vi "Autosampler Priming Settings Dialog.vi"(8 "error in":errorcluster, 10 "Valve Pos Names":string[](array[string])) -> (0 "error out":errorcluster, 1 "Cancelled?":bool, 2 "Result":T1)   [LabVIEW 2023]
panel:
  in  "Output Valve Position":u16(ring)=1 items=["1. Needle port", "2. Waste", "3. Disconnected", "4. Disconnected", "5. Disconnected", "6. Water"]
  in  "Input Valve Position":u16(ring)=5 items=["1. Needle port", "2. Waste", "3. Disconnected", "4. Disconnected", "5. Disconnected", "6. Water"]
  in  "Cancel":bool caption="Boolean 2"
  in  "Ok":bool caption="Boolean"
  in  "Number of Cycles":u16=3 min=1 step=1
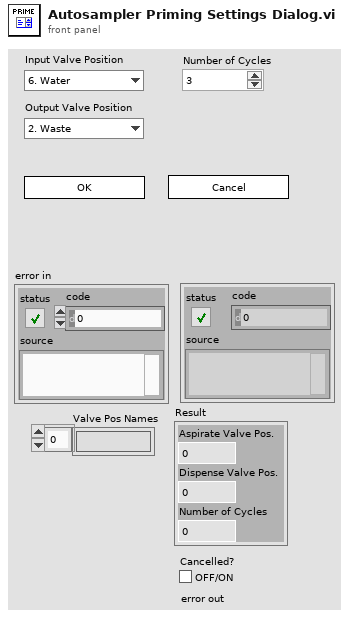
[diagram p1: front panel]
types:
  T1 = cluster{"Aspirate Valve Pos.":u16, "Dispense Valve Pos.":u16, "Number of Cycles":u16}
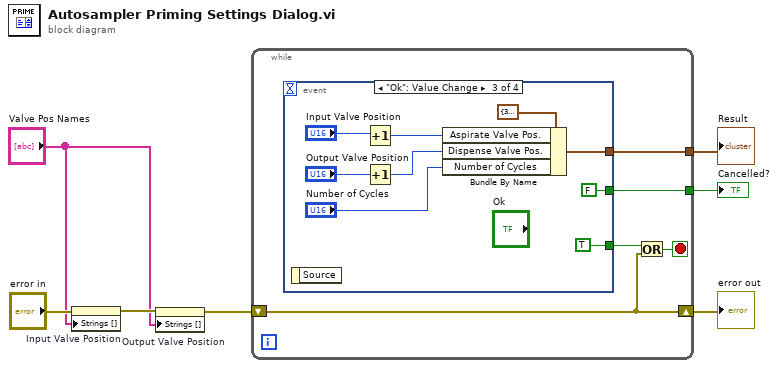
[diagram p0: block diagram]
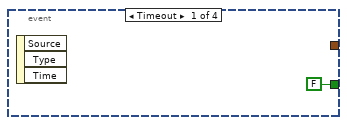
[diagram p2: hidden frame]
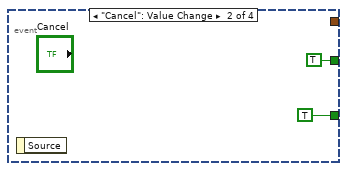
[diagram p3: hidden frame]
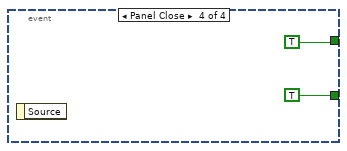
[diagram p4: hidden frame]
diagram:
  n1 = property on="Input Valve Position" class="Ring (strict)"(error in="error in", "Strings []"="Valve Pos Names") -> (error out=w3:errorcluster)  [unwired: 1 in, 1 out]
  n2 = property on="Output Valve Position" class="Ring (strict)"(error in=w3, "Strings []"="Valve Pos Names") -> (error out=w2:errorcluster)  [unwired: 1 in, 1 out]
  n3 = while {
    shift-right: [w8] -> w7
    shift-left: w2 -> [w8]
    tunnel: [w12] -> w6
    tunnel: [w11] -> w5
    stop <- w10 stop-if-true
    n4 = event shown="[2] \"Ok\": Value Change" {
      selector: _ -> [_ _ _ _]
      dyn-events: _ -> [_ _ _ _]
      timeout: _ -> [_ _ _ _]
      tunnel: [FALSE TRUE FALSE TRUE] -> w12
      tunnel: [_ _ w21 _] -> w11
      tunnel: [_ TRUE TRUE TRUE] -> w9
      event Timeout {
        n5 = event-data() -> ()  [unwired: 1 in, 3 out]
      }
      event "Cancel": Value Change {
        n6 = event-data() -> ()  [unwired: 1 in, 1 out]
      }
      event "Ok": Value Change {
        n7 = event-data() -> ()  [unwired: 1 in, 1 out]
        n8 = Increment(x="Input Valve Position") -> (x+1=w18:u16)
        n9 = Increment(x="Output Valve Position") -> (x+1=w16:u16)
        n10 = Bundle By Name(cluster=T1 {"Aspirate Valve Pos."=3, "Dispense Valve Pos."=2, "Number of Cycles"=5}, "Aspirate Valve Pos."=w18, "Dispense Valve Pos."=w16, "Number of Cycles"="Number of Cycles") -> (w21:T1)
      }
      event Panel Close {
        n11 = event-data() -> ()  [unwired: 1 in, 1 out]
      }
    }
    n12 = Or(x=w9, y=w8) -> (x .or. y?=w10:bool)
  }
  "error out" <- w7
  "Cancelled?" <- w6
  "Result" <- w5
